vi "Abort Leaf Action.vi"(8 "error in (no error)":errorcluster, 11 "Root Actor in":refnum<class "Root Actor.lvclass">) -> (0 "error out":errorcluster, 3 "Root Actor out":refnum<class "Root Actor.lvclass">)   [LabVIEW 2019, in "Root Actor.lvclass"]
uses:
  Root Actor.lvclass
  Root Actor.lvclass/Root Actor.ctl
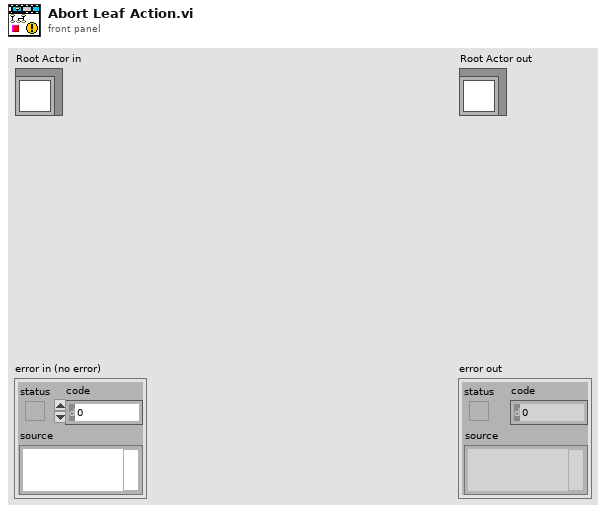
[diagram p1: front panel]
types:
  T1 = typedef "System Actor Stop Notifier.ctl" = refnum<notifier>
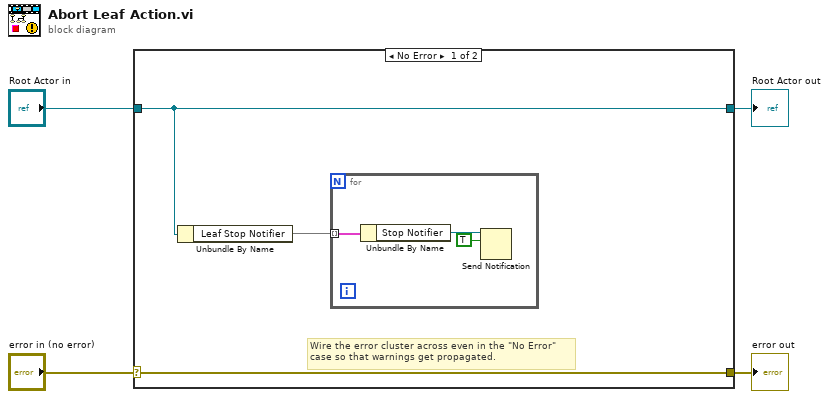
[diagram p0: block diagram]
diagram:
  n1 = case shown="No Error" "error in (no error)" {
    selector: "error in (no error)" -> [w7 w12]
    tunnel: [w7 w12] -> w3
    tunnel: [w5 w11] -> w1
    tunnel: "Root Actor in" -> [w5 w11]
    frame No Error {
      # "Wire the error cluster across even in the \"No Error\"\ncase so that warnings get propagated."
      n2 = Unbundle By Name(w5) -> ("Leaf Stop Notifier"=w6:map{i64[], T1})
      n3 = for {
        tunnel: w6 -> [w10] mode=indexing
        n4 = Unbundle By Name(w10) -> ("Stop Notifier"=w8:T1)
        n5 = Send Notification(notification=TRUE, notifier=w8) -> ()  [unwired: 1 in, 2 out]
      }
    }
    frame Error {
    }
  }
  "error out" <- w3
  "Root Actor out" <- w1
